vi "setResolutionInDigits.vi"(8 "error in (no error)":errorcluster, 10 "Digits":dbl, 11 "DmmKeysight in":refnum<class "DmmKeysight.lvclass">) -> (0 "error out":errorcluster, 3 "DmmKeysight out":refnum<class "DmmKeysight.lvclass">)   [LabVIEW 2023, in "DmmKeysight.lvclass"]
doc: "<b>Author:</b> Wolfgang\n<b>Description:</b> set multimeter resolution in digits 4.5, 5.5, 6.5"
uses:
  DmmKeysight.lvclass
  DmmKeysight.lvclass/DmmKeysight.ctl
  Multimeter.lvclass
  Driver/Keysight-34450A.lvlib
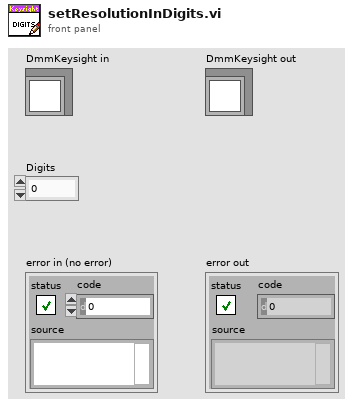
[diagram p1: front panel]
types:
  T1 = typedef "Keysight-34450A.lvlib/configuration.ctl" = cluster{"mode":T2, "Range":dbl, "Resolution":dbl}
  T2 = typedef "Keysight-34450A.lvlib/mode.ctl" = enum16{"DC_Voltage", "AC_Voltage", "DC_Current", "AC_Current", "Resistance"}
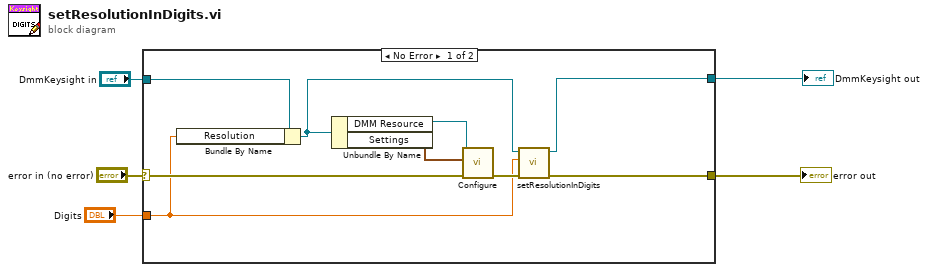
[diagram p0: block diagram]
diagram:
  n1 = case shown="No Error" "error in (no error)" {
    selector: "error in (no error)" -> [w7 w16]
    tunnel: [w14 w16] -> w5
    tunnel: [w13 w15] -> w4
    tunnel: "DmmKeysight in" -> [w12 w15]
    tunnel: "Digits" -> [w6 _]
    frame No Error {
      n2 = Bundle By Name(cluster=w12, "Resolution"=w6) -> (w10:refnum<class "DmmKeysight.lvclass">)
      n3 = Unbundle By Name(w10) -> ("DMM Resource"=w11:refnum<visa-resource-name>, "Settings"=w9:T1)
      n4 = call "Configure.vi"("error in (no error)"=w7, "Configuration"=w9, "VISA resource name"=w11) -> ("error out"=w8:errorcluster)  [unwired: 7 in, 1 out]
      n5 = call-parent "setResolutionInDigits.vi"("error in (no error)"=w8, "Resolution"=w6, "Multimeter in"=w10) -> ("error out"=w14:errorcluster, "Multimeter out"=w13:refnum<class "DmmKeysight.lvclass">)  [unwired: 7 in]
    }
    frame Error {
    }
  }
  "error out" <- w5
  "DmmKeysight out" <- w4
